vi "Autonomous Independent.vi"() -> ()   [LabVIEW 2016]
doc: "This VI is called when autonomous begins, and will automatically be terminated when autonomous ends. You can carry out timed or sensor driven robot movement independently without needing to return to the caller."
uses:
  <vilib>/Rock Robotics/WPI/SafetyOutput/WPI_SafetyOutputConfigMenu.ctl
  <vilib>/Rock Robotics/WPI/Utilities/WPI_GetSetVariantRefNum.vi
  <vilib>/Rock Robotics/Network Tables/NT Write Numeric Array.vi
panel:
  in  "Distance 3":dbl=64.0
  in  "Effort 3":dbl=-0.25 format="%#_13g"
  in  "Effort 2":dbl=-0.2 format="%#_13g"
  in  "Distance 2":dbl=77.544
  in  "Angle":dbl=55.0
  in  "Distance 1":dbl=54.0
  in  "Effort 1":dbl=-0.25 format="%#_13g"
  # "Be sure to right-click and choose Data Operations>>Make Current Value default if you want to save the array values with the VI"
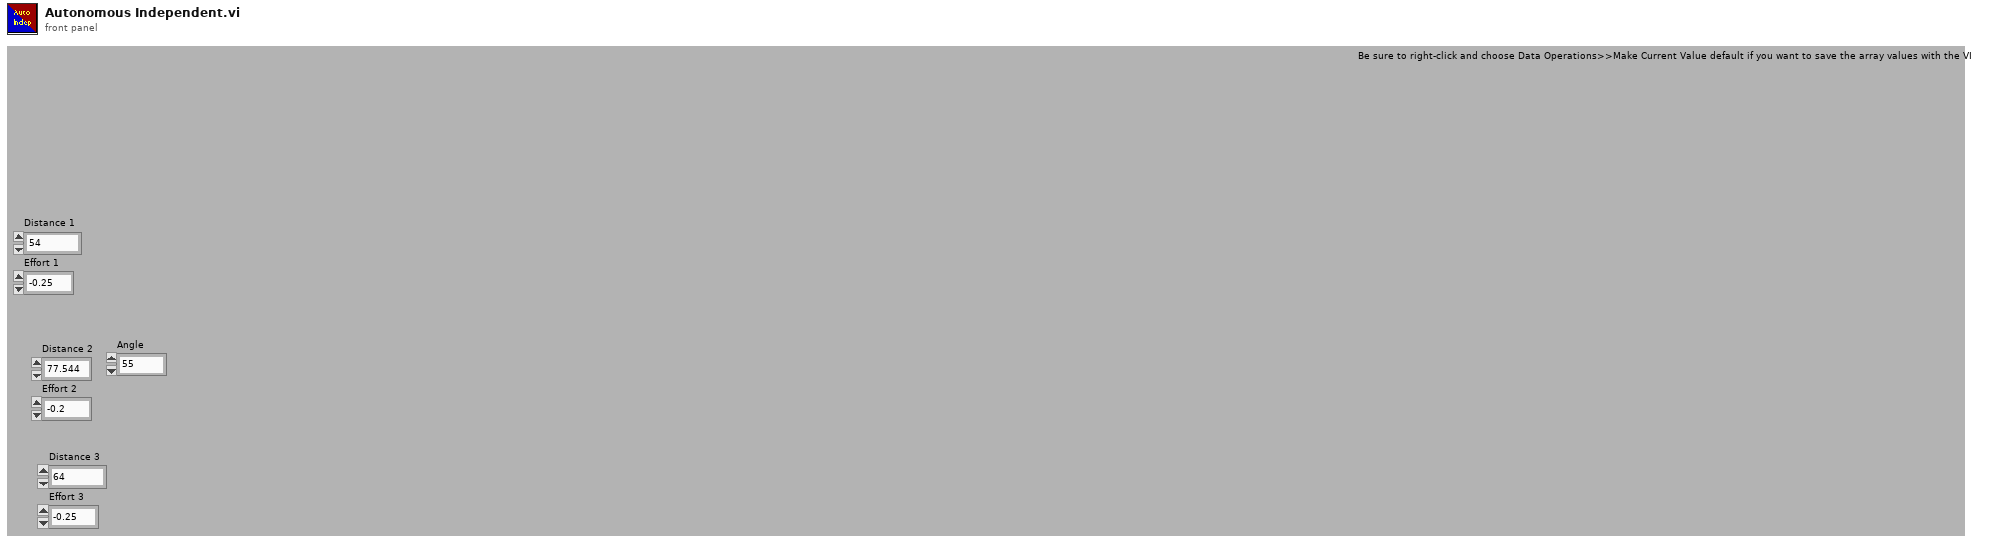
[diagram p1: front panel]
types:
  T1 = typedef "WPI_JoystickDevRef.ctl" = cluster{"Device":T2}
  T2 = typedef "WPI_JoystickDeviceEnum.ctl" = enum16{"USB 0", "USB 1", "USB 2", "USB 3", "USB 4", "USB 5"}
  T3 = typedef "WPI_SafetyOutputConfigMenu.ctl" = enum16{"Enable", "Disable"}
  T4 = typedef "WPI_MotorControlDeviceRef.ctl" = cluster{"DeviceStatus":errorcluster, "Type":T5, "PWM":cluster{"PWM Channel":T6, "DeadBand":T7}, "CAN":cluster{"Device Number":u8, "SetOutput VI Ref":variant, "GetOutput VI Ref":variant, "Enable VI Ref":variant, "Disable VI Ref":variant, "Data":variant}, "Invert":bool}
  T5 = typedef "WPI_MotorControlType.ctl" = enum16{"PWM", "CAN"}
  T6 = typedef "FPGA_DIOPWMChannel.ctl" = enum8{"PWM 0", "PWM 1", "PWM 2", "PWM 3", "PWM 4", "PWM 5", "PWM 6", "PWM 7", "PWM 8", "PWM 9", "PWM MXP 0", "PWM MXP 1", "PWM MXP 2", "PWM MXP 3", "PWM MXP 4", "PWM MXP 5", "PWM MXP 6", "PWM MXP 7", "PWM MXP 8", "PWM MXP 9", "Invalid"}
  T7 = typedef "WPI_PWMDeadband.ctl" = cluster{"Name":string, "maxPositivePwm":i32, "minPositivePwm":i32, "centerPwm":i32, "maxNegativePwm":i32, "minNegativePwm":i32, "angularRange":u16}
  T8 = typedef "WPI_CANTalonSRX_GlobalStatus.ctl" = cluster{"Applied Throttle":dbl, "Module Enabled":bool, "CAN Error":errorcluster, "Closed Loop Error":dbl, "Forward Limit Switch Closed":bool, "Reverse Limit Switch Closed":bool, "Sensor Position":dbl, "Sensor Velocity":dbl, "Current":dbl, "Sticky Fault - Over Temp":bool, "Sticky Fault - Under Voltage":bool, "Sticky Fault - Forward Limit":bool, "Sticky Fault - Reverse Limit":bool, "Sticky Fault - Forward Soft Limit":bool, "Sticky Fault - Reverse Soft Limit":bool, "Brake is Enabled":bool, "Encoder Position":dbl, "Encoder Velocity":dbl, "Encoder Index Count":dbl, "Encoder A Pin State":bool, "Encoder B Pin State":bool, "Encoder Index Pin State":bool, "Analog In":dbl, "Analog In Velocity":dbl, "Temperature (C)":dbl, "Battery Voltage":dbl, "Control 5 Is Supported":bool, "Current Profile Slot Select":dbl, "Pos Div 8":bool, "Vel Div 4":bool, "Pulse Width Position":i32, "Pulse Width Velocity":i32, "Pulse Width Rise To Rise (us)":i32, "Pulse Width Rise To Fall (us)":i32, "Mot Prof Active Is Under Run":bool, "Mot Prof Active Has Under Run":bool, "Mot Prof Active Is Last":bool, "Mot Prof Active Velocity Only":bool, "Mot Prof Active Is Valid":bool, "Mot Prof Buffer Is Full":bool, "Mot Prof Active Profile Slot Select":i32, "Mot Prof NextID":i32, "Mot Prof Count":i32, "Mot Prof Active Velocity":dbl, "Mot Prof Active Position":dbl, "Mot Prof Output Enable":i32}
  T9 = typedef "WPI_GyroDevRef.ctl" = cluster{"DevStatus":errorcluster, "Analog Channel":T10, "Offset":dbl, "Gain (VoltsPerDegree/Second)":dbl, "Gyro Type":enum16{"Analog", "XRS450"}, "Handle":i32, "SPI Bus":T11, "Device Found":bool, "Sample Rate":dbl, "Calibrate On Open":bool}
  T10 = typedef "FPGA_AIChannel.ctl" = enum8{"AI 0", "AI 1", "AI 2", "AI 3", "AI MXP 0", "AI MXP 1", "AI MXP 2", "AI MXP 3", "Invalid"}
  T11 = typedef "spi_bus.ctl" = enum16{"SPI On-Board, CS0", "SPI On-Board, CS1", "SPI On-Board, CS2", "SPI On-Board, CS3", "SPI MXP", "Invalid"}
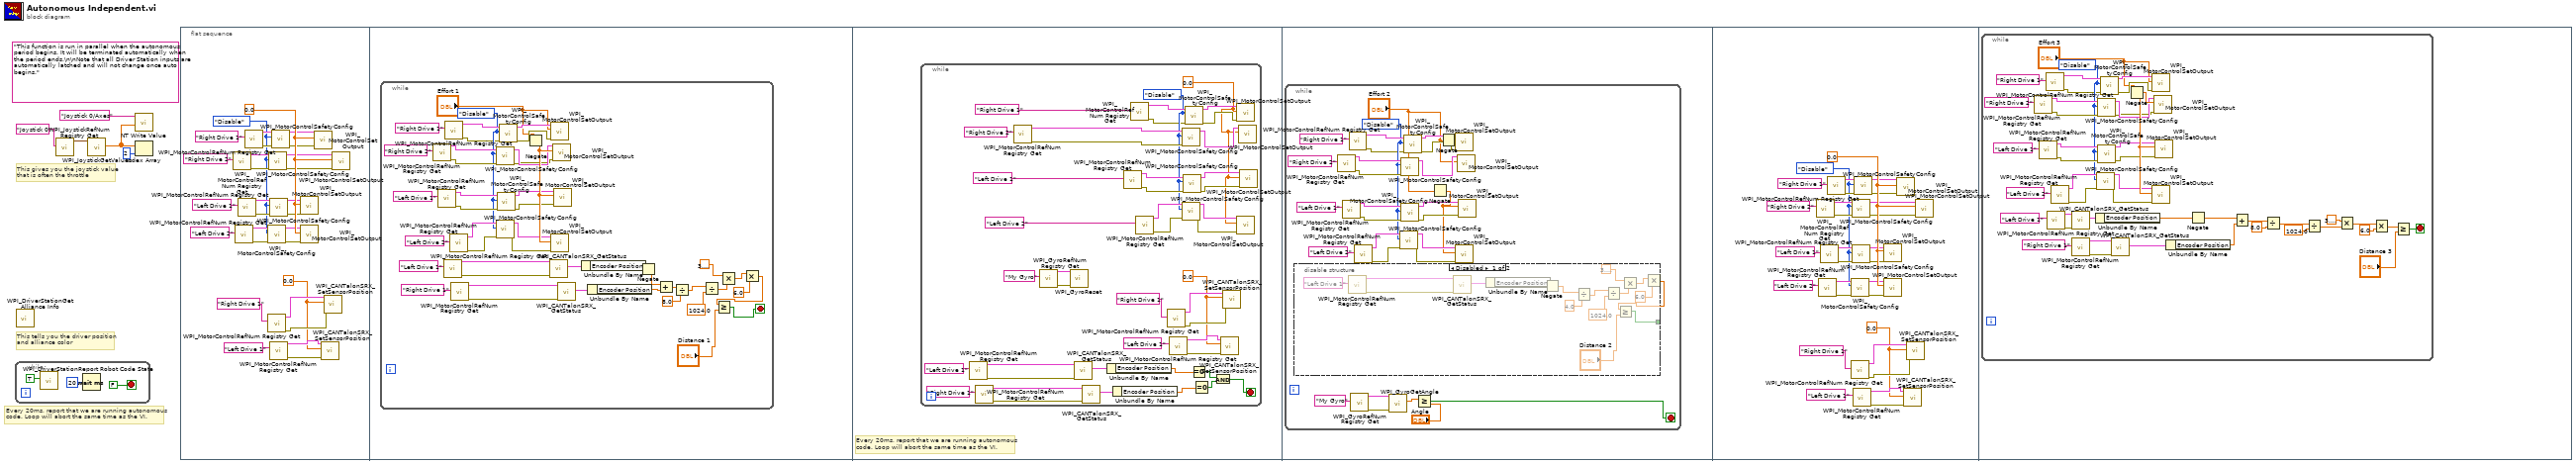
[diagram p0: block diagram]
diagram:
  (unwired) "This function is run in parallel when the autonomous period begins. It will be terminated automatically when the period ends.\n\nNote that all Driver Station inputs are automatically latched and will not change once auto begins."
  # "Every 20ms, report that we are running autonomous\ncode. Loop will abort the same time as the VI."
  # "This gives you the joystick value\nthat is often the throttle"
  # "This tells you the driver position\nand alliance color"
  n1 = while {
    stop <- FALSE stop-if-true
    n2 = call <vilib>:"WPI_DriverStationReport Robot Code State.vi"("Autonomous"=TRUE) -> ()  [unwired: 10 in, 1 out]
    n3 = Wait (ms)(milliseconds to wait=u32 20) -> ()  [unwired: 1 out]
  }
  n4 = call <vilib>:"WPI_DriverStationGet Alliance Info.vi"() -> ()  [unwired: 12 out]
  n5 = call <vilib>:"WPI_JoystickRefNum Registry Get.vi"("refnum name"="Joystick 0") -> ("JoystickDevRef"=w4:T1)  [unwired: 1 in, 9 out]
  n6 = call <vilib>:"WPI_JoystickGetValues.vi"("JoystickDevRef"=w4) -> ("Axes"=w2:dbl[])  [unwired: 6 in, 4 out]
  n7 = call-poly <vilib>:"NT Write Value.vi"("Numeric Array"=w2, "Name"="Joystick 0/Axes") -> ()  [unwired: 9 in, 1 out]
  n8 = Index Array(array=w2, index=2) -> ()  [unwired: 1 out]
  n9 = flat-sequence {
    frame #0 {
      w17 = WPI_SafetyOutputConfigMenu."Disable" ("mode")
      w26 = 0.0 ("Effort 2")
      w31 = 0.0 ("New Sensor Position")
      n10 = call <vilib>:"WPI_MotorControlRefNum Registry Get.vi"("refnum name"="Right Drive 2") -> ("error out"=w22:errorcluster, "MotorControlDevRef"=w23:T4)  [unwired: 9 in]
      n11 = call <vilib>:"WPI_MotorControlRefNum Registry Get.vi"("refnum name"="Left Drive 2") -> ("error out"=w18:errorcluster, "MotorControlDevRef"=w19:T4)  [unwired: 9 in]
      n12 = call <vilib>:"WPI_MotorControlRefNum Registry Get.vi"("refnum name"="Left Drive 1") -> ("error out"=w20:errorcluster, "MotorControlDevRef"=w21:T4)  [unwired: 9 in]
      n13 = call <vilib>:"WPI_MotorControlRefNum Registry Get.vi"("refnum name"="Right Drive 1") -> ("error out"=w25:errorcluster, "MotorControlDevRef"=w24:T4)  [unwired: 9 in]
      n14 = call <vilib>:"WPI_MotorControlSafetyConfig.vi"("error in (no error)"=w18, "mode"=w17, "MotorControlDevRef"=w19) -> ("error out"=w9:errorcluster, "MotorControlDevRef"=w10:T4)  [unwired: 7 in]
      n15 = call <vilib>:"WPI_MotorControlRefNum Registry Get.vi"("refnum name"="Right Drive 1") -> ("error out"=w32:errorcluster, "MotorControlDevRef"=w33:T4)  [unwired: 9 in]
      n16 = call <vilib>:"WPI_MotorControlSafetyConfig.vi"("error in (no error)"=w22, "mode"=w17, "MotorControlDevRef"=w23) -> ("error out"=w13:errorcluster, "MotorControlDevRef"=w14:T4)  [unwired: 7 in]
      n17 = call <vilib>:"WPI_MotorControlSafetyConfig.vi"("error in (no error)"=w20, "mode"=w17, "MotorControlDevRef"=w21) -> ("error out"=w11:errorcluster, "MotorControlDevRef"=w12:T4)  [unwired: 7 in]
      n18 = call <vilib>:"WPI_MotorControlRefNum Registry Get.vi"("refnum name"="Left Drive 1") -> ("error out"=w34:errorcluster, "MotorControlDevRef"=w35:T4)  [unwired: 9 in]
      n19 = call <vilib>:"WPI_MotorControlSafetyConfig.vi"("error in (no error)"=w25, "mode"=w17, "MotorControlDevRef"=w24) -> ("error out"=w15:errorcluster, "MotorControlDevRef"=w16:T4)  [unwired: 7 in]
      n20 = call <vilib>:"WPI_MotorControlSetOutput.vi"("error in (no error)"=w11, "Output"=w26, "MotorControlDevRef"=w12) -> ()  [unwired: 6 in, 3 out]
      n21 = call <vilib>:"WPI_MotorControlSetOutput.vi"("error in (no error)"=w9, "Output"=w26, "MotorControlDevRef"=w10) -> ()  [unwired: 6 in, 3 out]
      n22 = call <vilib>:"WPI_MotorControlSetOutput.vi"("error in (no error)"=w15, "Output"=w26, "MotorControlDevRef"=w16) -> ()  [unwired: 6 in, 3 out]
      n23 = call <vilib>:"WPI_CANTalonSRX_SetSensorPosition.vi"("error in (no error)"=w34, "New Sensor Position"=w31, "CAN Talon SRX Ref"=w35) -> ()  [unwired: 7 in, 2 out]
      n24 = call <vilib>:"WPI_CANTalonSRX_SetSensorPosition.vi"("error in (no error)"=w32, "New Sensor Position"=w31, "CAN Talon SRX Ref"=w33) -> ()  [unwired: 7 in, 2 out]
      n25 = call <vilib>:"WPI_MotorControlSetOutput.vi"("error in (no error)"=w13, "Output"=w26, "MotorControlDevRef"=w14) -> ()  [unwired: 6 in, 3 out]
    }
    frame #1 {
      n26 = while {
        stop <- w48 stop-if-true
        w54 = WPI_SafetyOutputConfigMenu."Disable" ("mode")
        n27 = call <vilib>:"WPI_MotorControlRefNum Registry Get.vi"("refnum name"="Right Drive 2") -> ("error out"=w57:errorcluster, "MotorControlDevRef"=w58:T4)  [unwired: 9 in]
        n28 = call <vilib>:"WPI_MotorControlRefNum Registry Get.vi"("refnum name"="Left Drive 1") -> ("error out"=w61:errorcluster, "MotorControlDevRef"=w62:T4)  [unwired: 9 in]
        n29 = call <vilib>:"WPI_MotorControlRefNum Registry Get.vi"("refnum name"="Left Drive 1") -> ("error out"=w81:errorcluster, "MotorControlDevRef"=w82:T4)  [unwired: 9 in]
        n30 = call <vilib>:"WPI_MotorControlRefNum Registry Get.vi"("refnum name"="Right Drive 1") -> ("error out"=w52:errorcluster, "MotorControlDevRef"=w69:T4)  [unwired: 9 in]
        n31 = call <vilib>:"WPI_MotorControlRefNum Registry Get.vi"("refnum name"="Left Drive 2") -> ("error out"=w65:errorcluster, "MotorControlDevRef"=w66:T4)  [unwired: 9 in]
        n32 = call <vilib>:"WPI_MotorControlRefNum Registry Get.vi"("refnum name"="Right Drive 1") -> ("error out"=w46:errorcluster, "MotorControlDevRef"=w80:T4)  [unwired: 9 in]
        n33 = call <vilib>:"WPI_MotorControlSafetyConfig.vi"("error in (no error)"=w65, "mode"=w54, "MotorControlDevRef"=w66) -> ("error out"=w63:errorcluster, "MotorControlDevRef"=w64:T4)  [unwired: 7 in]
        n34 = call <vilib>:"WPI_MotorControlSafetyConfig.vi"("error in (no error)"=w57, "mode"=w54, "MotorControlDevRef"=w58) -> ("error out"=w55:errorcluster, "MotorControlDevRef"=w56:T4)  [unwired: 7 in]
        n35 = call <vilib>:"WPI_MotorControlSafetyConfig.vi"("error in (no error)"=w61, "mode"=w54, "MotorControlDevRef"=w62) -> ("error out"=w59:errorcluster, "MotorControlDevRef"=w60:T4)  [unwired: 7 in]
        n36 = call <vilib>:"WPI_MotorControlSafetyConfig.vi"("error in (no error)"=w52, "mode"=w54, "MotorControlDevRef"=w69) -> ("error out"=w53:errorcluster, "MotorControlDevRef"=w68:T4)  [unwired: 7 in]
        n37 = Negate(x="Effort 1") -> (-x=w67:dbl)
        n38 = call <vilib>:"WPI_CANTalonSRX_GetStatus.vi"("error in (no error)"=w81, "CAN Talon SRX Ref"=w82) -> ("Talon SRX Status"=w38:T8)  [unwired: 7 in, 2 out]
        n39 = call <vilib>:"WPI_MotorControlSetOutput.vi"("error in (no error)"=w53, "Output"="Effort 1", "MotorControlDevRef"=w68) -> ()  [unwired: 6 in, 3 out]
        n40 = call <vilib>:"WPI_MotorControlSetOutput.vi"("error in (no error)"=w63, "Output"=w67, "MotorControlDevRef"=w64) -> ()  [unwired: 6 in, 3 out]
        n41 = call <vilib>:"WPI_MotorControlSetOutput.vi"("error in (no error)"=w55, "Output"=w67, "MotorControlDevRef"=w56) -> ()  [unwired: 6 in, 3 out]
        n42 = call <vilib>:"WPI_MotorControlSetOutput.vi"("error in (no error)"=w59, "Output"=w67, "MotorControlDevRef"=w60) -> ()  [unwired: 6 in, 3 out]
        n43 = call <vilib>:"WPI_CANTalonSRX_GetStatus.vi"("error in (no error)"=w46, "CAN Talon SRX Ref"=w80) -> ("Talon SRX Status"=w50:T8)  [unwired: 7 in, 2 out]
        n44 = Unbundle By Name(w38) -> ("Encoder Position"=w72:dbl)
        n45 = Unbundle By Name(w50) -> ("Encoder Position"=w73:dbl)
        n46 = Negate(x=w72) -> (-x=w49:dbl)
        n47 = Add(x=w49, y=w73) -> (x+y=w71:dbl)
        n48 = Divide(x=w71, y=8.0) -> (x/y=w45:dbl)
        n49 = Divide(x=w45, y=1024.0) -> (x/y=w42:dbl)
        n50 = Multiply(x=3.141592653589793, y=w42) -> (x*y=w43:dbl)
        n51 = Multiply(x=w43, y=6.0) -> (x*y=w39:dbl)
        n52 = Greater Or Equal?(x=w39, y="Distance 1") -> (x >= y?=w48:bool)
      }
    }
    frame #2 {
      # "Every 20ms, report that we are running autonomous\ncode. Loop will abort the same time as the VI."
      n53 = while {
        stop <- w86 stop-if-true
        w99 = 0.0
        w103 = WPI_SafetyOutputConfigMenu."Disable" ("mode")
        w120 = 0.0 ("New Sensor Position")
        n54 = call <vilib>:"WPI_MotorControlRefNum Registry Get.vi"("refnum name"="Left Drive 1") -> ("error out"=w97:errorcluster, "MotorControlDevRef"=w98:T4)  [unwired: 9 in]
        n55 = call <vilib>:"WPI_MotorControlRefNum Registry Get.vi"("refnum name"="Right Drive 1") -> ("error out"=w91:errorcluster, "MotorControlDevRef"=w95:T4)  [unwired: 9 in]
        n56 = call <vilib>:"WPI_MotorControlRefNum Registry Get.vi"("refnum name"="Right Drive 2") -> ("error out"=w104:errorcluster, "MotorControlDevRef"=w105:T4)  [unwired: 9 in]
        n57 = call <vilib>:"WPI_GyroRefNum Registry Get.vi"("refnum name"="My Gyro") -> ("error out"=w84:errorcluster, "GyroDevRef"=w83:T9)  [unwired: 9 in]
        n58 = call <vilib>:"WPI_GyroReset.vi"("error in"=w84, "GyroDevRef"=w83) -> ()  [unwired: 8 in, 2 out]
        n59 = call <vilib>:"WPI_CANTalonSRX_GetStatus.vi"("error in (no error)"=w97, "CAN Talon SRX Ref"=w98) -> ("Talon SRX Status"=w96:T8)  [unwired: 7 in, 2 out]
        n60 = call <vilib>:"WPI_CANTalonSRX_GetStatus.vi"("error in (no error)"=w91, "CAN Talon SRX Ref"=w95) -> ("Talon SRX Status"=w92:T8)  [unwired: 7 in, 2 out]
        n61 = Unbundle By Name(w96) -> ("Encoder Position"=w90:dbl)
        n62 = Unbundle By Name(w92) -> ("Encoder Position"=w88:dbl)
        n63 = call <vilib>:"WPI_MotorControlRefNum Registry Get.vi"("refnum name"="Left Drive 1") -> ("error out"=w108:errorcluster, "MotorControlDevRef"=w109:T4)  [unwired: 9 in]
        n64 = call <vilib>:"WPI_MotorControlRefNum Registry Get.vi"("refnum name"="Right Drive 1") -> ("error out"=w101:errorcluster, "MotorControlDevRef"=w115:T4)  [unwired: 9 in]
        n65 = call <vilib>:"WPI_MotorControlRefNum Registry Get.vi"("refnum name"="Left Drive 2") -> ("error out"=w112:errorcluster, "MotorControlDevRef"=w113:T4)  [unwired: 9 in]
        n66 = call <vilib>:"WPI_MotorControlRefNum Registry Get.vi"("refnum name"="Right Drive 1") -> ("error out"=w121:errorcluster, "MotorControlDevRef"=w122:T4)  [unwired: 9 in]
        n67 = call <vilib>:"WPI_MotorControlRefNum Registry Get.vi"("refnum name"="Left Drive 1") -> ("error out"=w123:errorcluster, "MotorControlDevRef"=w124:T4)  [unwired: 9 in]
        n68 = call <vilib>:"WPI_MotorControlSafetyConfig.vi"("error in (no error)"=w112, "mode"=w103, "MotorControlDevRef"=w113) -> ("error out"=w110:errorcluster, "MotorControlDevRef"=w111:T4)  [unwired: 7 in]
        n69 = call <vilib>:"WPI_MotorControlSafetyConfig.vi"("error in (no error)"=w104, "mode"=w103, "MotorControlDevRef"=w105) -> ("MotorControlDevRef"=w100:T4)  [unwired: 7 in, 1 out]
        n70 = call <vilib>:"WPI_MotorControlSafetyConfig.vi"("error in (no error)"=w108, "mode"=w103, "MotorControlDevRef"=w109) -> ("error out"=w106:errorcluster, "MotorControlDevRef"=w107:T4)  [unwired: 7 in]
        n71 = call <vilib>:"WPI_MotorControlSafetyConfig.vi"("error in (no error)"=w101, "mode"=w103, "MotorControlDevRef"=w115) -> ("error out"=w102:errorcluster, "MotorControlDevRef"=w114:T4)  [unwired: 7 in]
        n72 = Equal To 0?(x=w90) -> (x = 0?=w89:bool)
        n73 = Equal To 0?(x=w88) -> (x = 0?=w87:bool)
        n74 = And(x=w89, y=w87) -> (x .and. y?=w86:bool)
        n75 = call <vilib>:"WPI_CANTalonSRX_SetSensorPosition.vi"("error in (no error)"=w123, "New Sensor Position"=w120, "CAN Talon SRX Ref"=w124) -> ()  [unwired: 7 in, 2 out]
        n76 = call <vilib>:"WPI_CANTalonSRX_SetSensorPosition.vi"("error in (no error)"=w121, "New Sensor Position"=w120, "CAN Talon SRX Ref"=w122) -> ()  [unwired: 7 in, 2 out]
        n77 = call <vilib>:"WPI_MotorControlSetOutput.vi"("error in (no error)"=w102, "Output"=w99, "MotorControlDevRef"=w114) -> ()  [unwired: 6 in, 3 out]
        n78 = call <vilib>:"WPI_MotorControlSetOutput.vi"("error in (no error)"=w110, "Output"=w99, "MotorControlDevRef"=w111) -> ()  [unwired: 6 in, 3 out]
        n79 = call <vilib>:"WPI_MotorControlSetOutput.vi"("Output"=w99, "MotorControlDevRef"=w100) -> ()  [unwired: 7 in, 3 out]
        n80 = call <vilib>:"WPI_MotorControlSetOutput.vi"("error in (no error)"=w106, "Output"=w99, "MotorControlDevRef"=w107) -> ()  [unwired: 6 in, 3 out]
      }
    }
    frame #3 {
      n81 = while {
        stop <- w129 stop-if-true
        w139 = WPI_SafetyOutputConfigMenu."Disable" ("mode")
        n82 = disable-structure shown="Disabled" {
          disable-tunnel: [w165 _] -> _
          frame Disabled {
            n83 = call <vilib>:"WPI_MotorControlRefNum Registry Get.vi"("refnum name"="Left Drive 1") -> ("error out"=w170:errorcluster, "MotorControlDevRef"=w171:T4)  [unwired: 9 in]
            n84 = call <vilib>:"WPI_CANTalonSRX_GetStatus.vi"("error in (no error)"=w170, "CAN Talon SRX Ref"=w171) -> ("Talon SRX Status"=w169:T8)  [unwired: 7 in, 2 out]
            n85 = Unbundle By Name(w169) -> ("Encoder Position"=w167:dbl)
            n86 = Negate(x=w167) -> (-x=w157:dbl)
            n87 = Divide(x=w157, y=4.0) -> (x/y=w163:dbl)
            n88 = Divide(x=w163, y=1024.0) -> (x/y=w161:dbl)
            n89 = Multiply(x=3.141592653589793, y=w161) -> (x*y=w162:dbl)
            n90 = Multiply(x=w162, y=6.0) -> (x*y=w158:dbl)
            n91 = Greater Or Equal?(x=w158, y="Distance 2") -> (x >= y?=w165:bool)
          }
          frame Enabled {
          }
        }
        n92 = call <vilib>:"WPI_MotorControlRefNum Registry Get.vi"("refnum name"="Right Drive 2") -> ("error out"=w140:errorcluster, "MotorControlDevRef"=w141:T4)  [unwired: 9 in]
        n93 = call <vilib>:"WPI_MotorControlRefNum Registry Get.vi"("refnum name"="Left Drive 1") -> ("error out"=w144:errorcluster, "MotorControlDevRef"=w145:T4)  [unwired: 9 in]
        n94 = call <vilib>:"WPI_MotorControlRefNum Registry Get.vi"("refnum name"="Right Drive 1") -> ("error out"=w137:errorcluster, "MotorControlDevRef"=w151:T4)  [unwired: 9 in]
        n95 = call <vilib>:"WPI_GyroRefNum Registry Get.vi"("refnum name"="My Gyro") -> ("error out"=w134:errorcluster, "GyroDevRef"=w133:T9)  [unwired: 9 in]
        n96 = call <vilib>:"WPI_MotorControlRefNum Registry Get.vi"("refnum name"="Left Drive 2") -> ("error out"=w148:errorcluster, "MotorControlDevRef"=w149:T4)  [unwired: 9 in]
        n97 = call <vilib>:"WPI_GyroGetAngle.vi"("error in"=w134, "GyroDevRef"=w133) -> ("Angle"=w131:dbl)  [unwired: 5 in, 4 out]
        n98 = call <vilib>:"WPI_MotorControlSafetyConfig.vi"("error in (no error)"=w148, "mode"=w139, "MotorControlDevRef"=w149) -> ("error out"=w146:errorcluster, "MotorControlDevRef"=w147:T4)  [unwired: 7 in]
        n99 = call <vilib>:"WPI_MotorControlSafetyConfig.vi"("error in (no error)"=w140, "mode"=w139, "MotorControlDevRef"=w141) -> ("MotorControlDevRef"=w136:T4)  [unwired: 7 in, 1 out]
        n100 = call <vilib>:"WPI_MotorControlSafetyConfig.vi"("error in (no error)"=w144, "mode"=w139, "MotorControlDevRef"=w145) -> ("error out"=w142:errorcluster, "MotorControlDevRef"=w143:T4)  [unwired: 7 in]
        n101 = call <vilib>:"WPI_MotorControlSafetyConfig.vi"("error in (no error)"=w137, "mode"=w139, "MotorControlDevRef"=w151) -> ("error out"=w138:errorcluster, "MotorControlDevRef"=w150:T4)  [unwired: 7 in]
        n102 = Greater Or Equal?(x=w131, y="Angle") -> (x >= y?=w129:bool)
        n103 = Negate(x="Effort 2") -> (-x=w135:dbl)
        n104 = Negate(x="Effort 2") -> (-x=w127:dbl)
        n105 = call <vilib>:"WPI_MotorControlSetOutput.vi"("error in (no error)"=w138, "Output"=w127, "MotorControlDevRef"=w150) -> ()  [unwired: 6 in, 3 out]
        n106 = call <vilib>:"WPI_MotorControlSetOutput.vi"("error in (no error)"=w146, "Output"=w135, "MotorControlDevRef"=w147) -> ()  [unwired: 6 in, 3 out]
        n107 = call <vilib>:"WPI_MotorControlSetOutput.vi"("Output"="Effort 2", "MotorControlDevRef"=w136) -> ()  [unwired: 7 in, 3 out]
        n108 = call <vilib>:"WPI_MotorControlSetOutput.vi"("error in (no error)"=w142, "Output"=w135, "MotorControlDevRef"=w143) -> ()  [unwired: 6 in, 3 out]
      }
    }
    frame #4 {
      w180 = WPI_SafetyOutputConfigMenu."Disable" ("mode")
      w189 = 0.0 ("Effort 2")
      w194 = 0.0 ("New Sensor Position")
      n109 = call <vilib>:"WPI_MotorControlRefNum Registry Get.vi"("refnum name"="Right Drive 2") -> ("error out"=w185:errorcluster, "MotorControlDevRef"=w186:T4)  [unwired: 9 in]
      n110 = call <vilib>:"WPI_MotorControlRefNum Registry Get.vi"("refnum name"="Left Drive 2") -> ("error out"=w181:errorcluster, "MotorControlDevRef"=w182:T4)  [unwired: 9 in]
      n111 = call <vilib>:"WPI_MotorControlRefNum Registry Get.vi"("refnum name"="Left Drive 1") -> ("error out"=w183:errorcluster, "MotorControlDevRef"=w184:T4)  [unwired: 9 in]
      n112 = call <vilib>:"WPI_MotorControlRefNum Registry Get.vi"("refnum name"="Right Drive 1") -> ("error out"=w188:errorcluster, "MotorControlDevRef"=w187:T4)  [unwired: 9 in]
      n113 = call <vilib>:"WPI_MotorControlSafetyConfig.vi"("error in (no error)"=w181, "mode"=w180, "MotorControlDevRef"=w182) -> ("error out"=w172:errorcluster, "MotorControlDevRef"=w173:T4)  [unwired: 7 in]
      n114 = call <vilib>:"WPI_MotorControlRefNum Registry Get.vi"("refnum name"="Right Drive 1") -> ("error out"=w195:errorcluster, "MotorControlDevRef"=w196:T4)  [unwired: 9 in]
      n115 = call <vilib>:"WPI_MotorControlSafetyConfig.vi"("error in (no error)"=w185, "mode"=w180, "MotorControlDevRef"=w186) -> ("error out"=w176:errorcluster, "MotorControlDevRef"=w177:T4)  [unwired: 7 in]
      n116 = call <vilib>:"WPI_MotorControlSafetyConfig.vi"("error in (no error)"=w183, "mode"=w180, "MotorControlDevRef"=w184) -> ("error out"=w174:errorcluster, "MotorControlDevRef"=w175:T4)  [unwired: 7 in]
      n117 = call <vilib>:"WPI_MotorControlRefNum Registry Get.vi"("refnum name"="Left Drive 1") -> ("error out"=w197:errorcluster, "MotorControlDevRef"=w198:T4)  [unwired: 9 in]
      n118 = call <vilib>:"WPI_MotorControlSafetyConfig.vi"("error in (no error)"=w188, "mode"=w180, "MotorControlDevRef"=w187) -> ("error out"=w178:errorcluster, "MotorControlDevRef"=w179:T4)  [unwired: 7 in]
      n119 = call <vilib>:"WPI_MotorControlSetOutput.vi"("error in (no error)"=w174, "Output"=w189, "MotorControlDevRef"=w175) -> ()  [unwired: 6 in, 3 out]
      n120 = call <vilib>:"WPI_MotorControlSetOutput.vi"("error in (no error)"=w172, "Output"=w189, "MotorControlDevRef"=w173) -> ()  [unwired: 6 in, 3 out]
      n121 = call <vilib>:"WPI_MotorControlSetOutput.vi"("error in (no error)"=w178, "Output"=w189, "MotorControlDevRef"=w179) -> ()  [unwired: 6 in, 3 out]
      n122 = call <vilib>:"WPI_CANTalonSRX_SetSensorPosition.vi"("error in (no error)"=w197, "New Sensor Position"=w194, "CAN Talon SRX Ref"=w198) -> ()  [unwired: 7 in, 2 out]
      n123 = call <vilib>:"WPI_CANTalonSRX_SetSensorPosition.vi"("error in (no error)"=w195, "New Sensor Position"=w194, "CAN Talon SRX Ref"=w196) -> ()  [unwired: 7 in, 2 out]
      n124 = call <vilib>:"WPI_MotorControlSetOutput.vi"("error in (no error)"=w176, "Output"=w189, "MotorControlDevRef"=w177) -> ()  [unwired: 6 in, 3 out]
    }
    frame #5 {
      n125 = while {
        stop <- w211 stop-if-true
        w217 = WPI_SafetyOutputConfigMenu."Disable" ("mode")
        n126 = call <vilib>:"WPI_MotorControlRefNum Registry Get.vi"("refnum name"="Right Drive 2") -> ("error out"=w220:errorcluster, "MotorControlDevRef"=w221:T4)  [unwired: 9 in]
        n127 = call <vilib>:"WPI_MotorControlRefNum Registry Get.vi"("refnum name"="Left Drive 1") -> ("error out"=w224:errorcluster, "MotorControlDevRef"=w225:T4)  [unwired: 9 in]
        n128 = call <vilib>:"WPI_MotorControlRefNum Registry Get.vi"("refnum name"="Right Drive 1") -> ("error out"=w215:errorcluster, "MotorControlDevRef"=w232:T4)  [unwired: 9 in]
        n129 = call <vilib>:"WPI_MotorControlRefNum Registry Get.vi"("refnum name"="Left Drive 1") -> ("error out"=w244:errorcluster, "MotorControlDevRef"=w245:T4)  [unwired: 9 in]
        n130 = call <vilib>:"WPI_MotorControlRefNum Registry Get.vi"("refnum name"="Left Drive 2") -> ("error out"=w228:errorcluster, "MotorControlDevRef"=w229:T4)  [unwired: 9 in]
        n131 = call <vilib>:"WPI_CANTalonSRX_GetStatus.vi"("error in (no error)"=w244, "CAN Talon SRX Ref"=w245) -> ("Talon SRX Status"=w201:T8)  [unwired: 7 in, 2 out]
        n132 = call <vilib>:"WPI_MotorControlRefNum Registry Get.vi"("refnum name"="Right Drive 1") -> ("error out"=w209:errorcluster, "MotorControlDevRef"=w243:T4)  [unwired: 9 in]
        n133 = Unbundle By Name(w201) -> ("Encoder Position"=w235:dbl)
        n134 = call <vilib>:"WPI_MotorControlSafetyConfig.vi"("error in (no error)"=w228, "mode"=w217, "MotorControlDevRef"=w229) -> ("error out"=w226:errorcluster, "MotorControlDevRef"=w227:T4)  [unwired: 7 in]
        n135 = call <vilib>:"WPI_MotorControlSafetyConfig.vi"("error in (no error)"=w220, "mode"=w217, "MotorControlDevRef"=w221) -> ("error out"=w218:errorcluster, "MotorControlDevRef"=w219:T4)  [unwired: 7 in]
        n136 = call <vilib>:"WPI_MotorControlSafetyConfig.vi"("error in (no error)"=w224, "mode"=w217, "MotorControlDevRef"=w225) -> ("error out"=w222:errorcluster, "MotorControlDevRef"=w223:T4)  [unwired: 7 in]
        n137 = call <vilib>:"WPI_MotorControlSafetyConfig.vi"("error in (no error)"=w215, "mode"=w217, "MotorControlDevRef"=w232) -> ("error out"=w216:errorcluster, "MotorControlDevRef"=w231:T4)  [unwired: 7 in]
        n138 = call <vilib>:"WPI_CANTalonSRX_GetStatus.vi"("error in (no error)"=w209, "CAN Talon SRX Ref"=w243) -> ("Talon SRX Status"=w213:T8)  [unwired: 7 in, 2 out]
        n139 = Negate(x="Effort 3") -> (-x=w230:dbl)
        n140 = call <vilib>:"WPI_MotorControlSetOutput.vi"("error in (no error)"=w216, "Output"="Effort 3", "MotorControlDevRef"=w231) -> ()  [unwired: 6 in, 3 out]
        n141 = call <vilib>:"WPI_MotorControlSetOutput.vi"("error in (no error)"=w226, "Output"=w230, "MotorControlDevRef"=w227) -> ()  [unwired: 6 in, 3 out]
        n142 = call <vilib>:"WPI_MotorControlSetOutput.vi"("error in (no error)"=w218, "Output"=w230, "MotorControlDevRef"=w219) -> ()  [unwired: 6 in, 3 out]
        n143 = call <vilib>:"WPI_MotorControlSetOutput.vi"("error in (no error)"=w222, "Output"=w230, "MotorControlDevRef"=w223) -> ()  [unwired: 6 in, 3 out]
        n144 = Unbundle By Name(w213) -> ("Encoder Position"=w236:dbl)
        n145 = Negate(x=w235) -> (-x=w212:dbl)
        n146 = Add(x=w212, y=w236) -> (x+y=w234:dbl)
        n147 = Divide(x=w234, y=8.0) -> (x/y=w208:dbl)
        n148 = Divide(x=w208, y=1024.0) -> (x/y=w205:dbl)
        n149 = Multiply(x=3.141592653589793, y=w205) -> (x*y=w206:dbl)
        n150 = Multiply(x=w206, y=6.0) -> (x*y=w202:dbl)
        n151 = Greater Or Equal?(x=w202, y="Distance 3") -> (x >= y?=w211:bool)
      }
    }
  }
